vi "Frequency_Response_Data_Smoothing_Shifting_mV.vi"(0 "smoothing":bool, 1 "curveShifting":bool, 2 "Parameters.RefAmplitude":dbl, 3 "Parameters.UUTResponseLevel.frequency":dbl[](array[numeric]), 4 "Parameters.UUTResponseLevel.amplitude":dbl[](array[numeric]), 5 "FG.FrequencyLists.FrequencyResponse_LimitHigh.amplitude":dbl[](array[numeric]), 7 "FG.FrequencyLists.FrequencyResponse_LimitLow.amplitude":dbl[](array[numeric])) -> (14 "ProcessedFrequencyResponse":dbl[](array[numeric]))   [LabVIEW 2018]
uses:
  <vilib>/Analysis/6fits.llb/Curve Fitting Criteria.ctl
  <vilib>/Analysis/6fits.llb/General Linear Fit Algorithm.ctl
  <vilib>/Analysis/NI_AALPro.lvlib
panel:
  out "XY Graph 2":cluster{dbl[], dbl[]}[](graph)
  out "max value":dbl=0.5912174990705221
  out "min value":dbl=2.180066627082418
  out "ShiftCurveBy":dbl=1.38564206307647
  out "XY Graph":cluster{dbl[], dbl[]}[](graph)
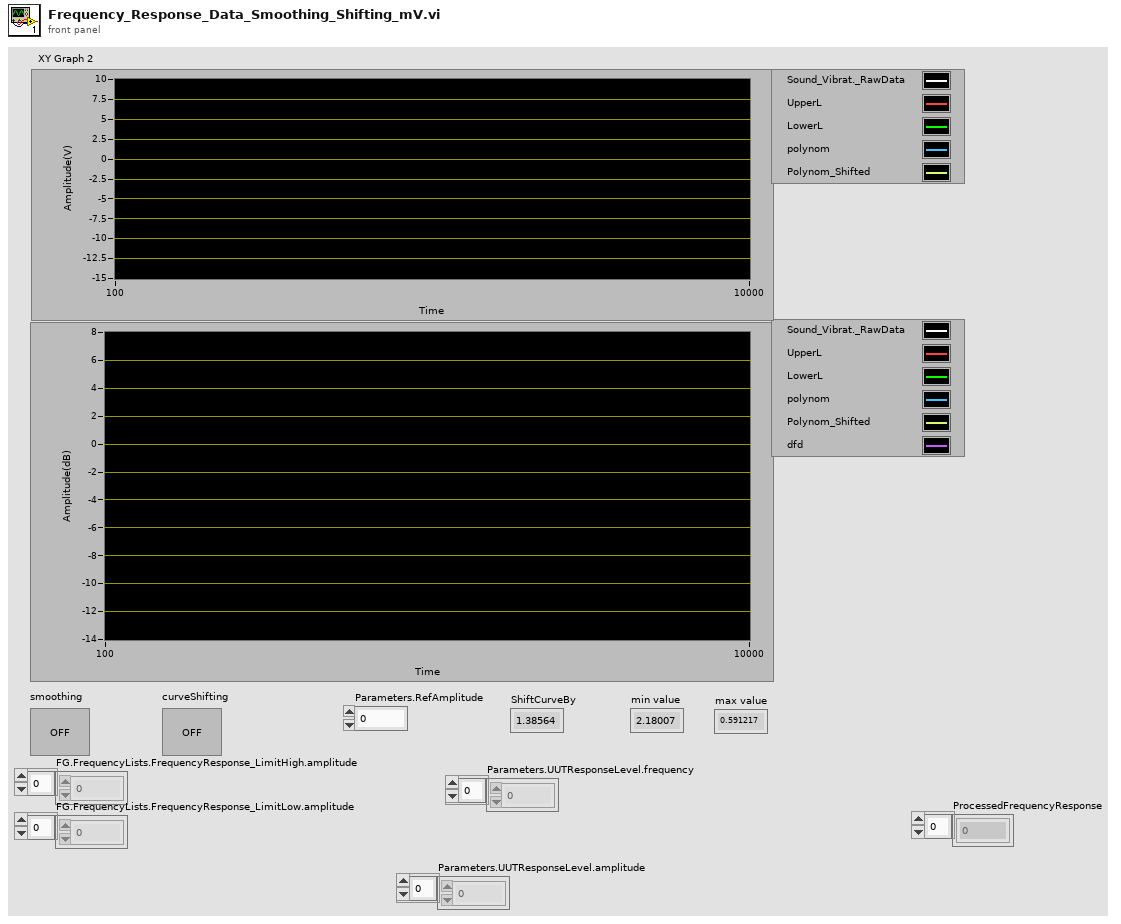
[diagram p1: front panel]
types:
  T1 = typedef "NI_AALPro.lvlib/General Linear Fit Algorithm.ctl" = u16
  T2 = typedef "NI_AALPro.lvlib/Curve Fitting Criteria.ctl" = u16
  T3 = cluster{"Parameters.UUTResponseLevel.frequency":dbl[], dbl[]}
  T4 = cluster{"Parameters.UUTResponseLevel.frequency":dbl[], dbl[]}[]
  T5 = cluster{"Parameters.UUTResponseLevel.frequency":dbl[], "FG.FrequencyLists.FrequencyResponse_LimitHigh.amplitude":dbl[]}
  T6 = cluster{"Parameters.UUTResponseLevel.frequency":dbl[], "FG.FrequencyLists.FrequencyResponse_LimitLow.amplitude":dbl[]}
  T7 = cluster{"Parameters.UUTResponseLevel.frequency":dbl[], "Best Polynomial Fit":dbl[]}
  T8 = cluster{"Parameters.UUTResponseLevel.frequency":dbl[], "Best Polynomial Fit":dbl[]}[]
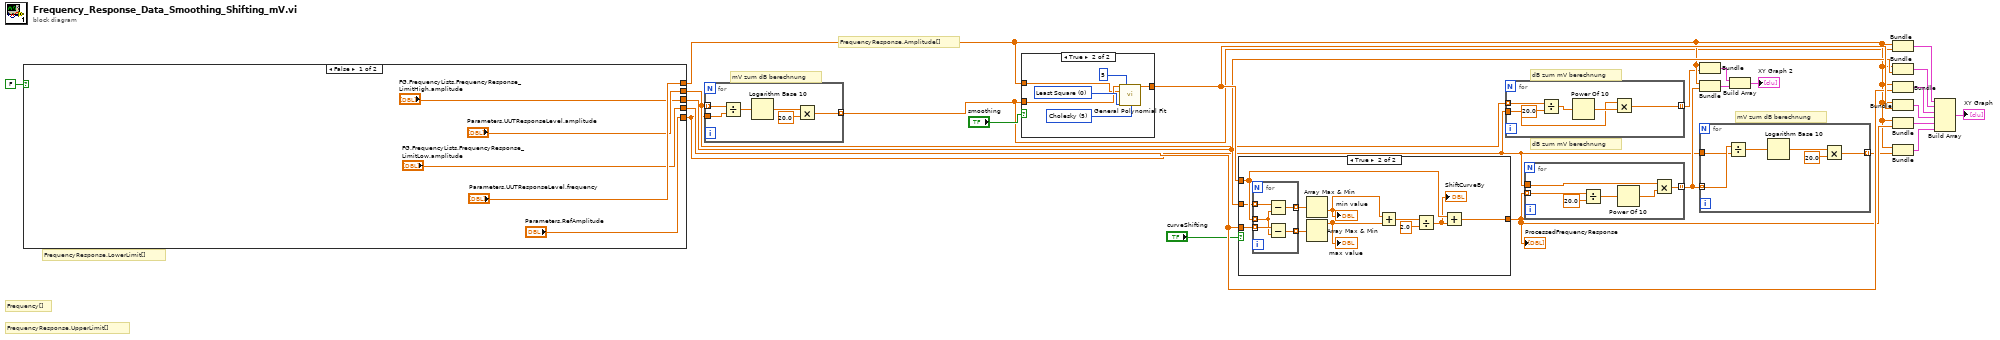
[diagram p0: block diagram]
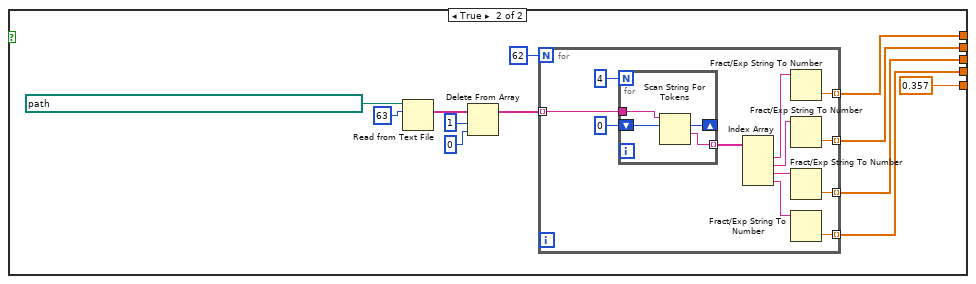
[diagram p2: hidden frame]
diagram:
  # "mV zum dB berechnung"
  # "mV zum dB berechnung"
  # "dB zum mV berechnung"
  # "dB zum mV berechnung"
  # "FrequencyResponse.LowerLimit[]"
  # "FrequencyResponse.UpperLimit[]"
  # "FrequencyResponse.Amplitude[]"
  # "Frequency[]"
  n1 = case shown="False" FALSE {
    tunnel: ["FG.FrequencyLists.FrequencyResponse_LimitLow.amplitude" w34] -> w17
    tunnel: ["FG.FrequencyLists.FrequencyResponse_LimitHigh.amplitude" w33] -> w16
    tunnel: ["Parameters.UUTResponseLevel.amplitude" w32] -> w3
    tunnel: ["Parameters.UUTResponseLevel.frequency" w31] -> w8
    tunnel: ["Parameters.RefAmplitude" 0.357 ("Parameters.RefAmplitude")] -> w2
    frame False {
    }
    frame True {
      n2 = Read from Text File(file (use dialog)=path "C:/Users/vr.ext/Desktop/Smoothing FG/SVT_Prüfstand_FG.txt", count=63) -> (text=w38:string[])  [unwired: 2 in, 3 out]
      n3 = Delete From Array(array=w38, length=1, index=0) -> (array with subset deleted=w35:string[])  [unwired: 1 out]
      n4 = for {
        N: 62 -> [_]
        tunnel: w35 -> [w51] mode=indexing
        tunnel: [w53] -> w31 mode=indexing
        tunnel: [w52] -> w32 mode=indexing
        tunnel: [w43] -> w33 mode=indexing
        tunnel: [w42] -> w34 mode=indexing
        n5 = for {
          N: 4 -> [_]
          tunnel: w51 -> [w56]
          shift-right: [w57] -> _
          shift-left: 0 ("count") -> [w55]
          tunnel: [w54] -> w49 mode=indexing
          n6 = Scan String For Tokens(8:w55, 9:w56) -> (1:w54:string, 2:w57:i32)  [unwired: 4 in, 2 out]
        }
        n7 = Index Array(array=w49) -> (element #1=w48:string, element #2=w47:string, element #3=w45:string, element #4=w44:string)  [unwired: 4 in]
        n8 = Fract/Exp String To Number(string=w48) -> (number=w53:dbl)  [unwired: 3 in, 1 out]
        n9 = Fract/Exp String To Number(string=w47) -> (number=w52:dbl)  [unwired: 3 in, 1 out]
        n10 = Fract/Exp String To Number(string=w45) -> (number=w43:dbl)  [unwired: 3 in, 1 out]
        n11 = Fract/Exp String To Number(string=w44) -> (number=w42:dbl)  [unwired: 3 in, 1 out]
      }
    }
  }
  n12 = for {
    tunnel: w3 -> [w62] mode=indexing
    tunnel: [w59] -> w1 mode=indexing
    tunnel: w2 -> [w58]
    n13 = Divide(x=w62, y=w58) -> (x/y=w61:dbl)
    n14 = Logarithm Base 10(1:w61) -> (0:w60:dbl)
    n15 = Multiply(x=w60, y=20.0) -> (x*y=w59:dbl)
  }
  n16 = case shown="True" "smoothing" {
    tunnel: w1 -> [w64 w67]
    tunnel: w8 -> [_ w66]
    tunnel: [w64 w65] -> w19
    frame False {
    }
    frame True {
      w69 = T1 5 items=["SVD", "Givens", "Givens2", "Householder", "LU Decomposition", "Cholesky", "SVD for Rank Deficient H"] ("algorithm")
      w70 = T2 0 items=["Least Square", "Least Absolute Residual", "Bisquare"] ("method")
      n17 = call <vilib>:"General Polynomial Fit.vi"("Y"=w67, "polynomial order"=5, "X"=w66, "method"=w70, "algorithm"=w69) -> ("Best Polynomial Fit"=w65:dbl[])  [unwired: 7 in, 3 out]
    }
  }
  n18 = case shown="True" "curveShifting" {
    tunnel: w19 -> [w71 w80]
    tunnel: [w71 w79] -> w11
    tunnel: w17 -> [_ w78]
    tunnel: w16 -> [_ w77]
    frame False {
    }
    frame True {
      n19 = for {
        tunnel: w77 -> [w87] mode=indexing
        tunnel: w80 -> [w84] mode=indexing
        tunnel: [w86] -> w82 mode=indexing
        tunnel: w78 -> [w85] mode=indexing
        tunnel: [w83] -> w81 mode=indexing
        n20 = Subtract(x=w87, y=w84) -> (x-y=w86:dbl)
        n21 = Subtract(x=w85, y=w84) -> (x-y=w83:dbl)
      }
      n22 = Array Max & Min(array=w82) -> (min value=w76:dbl)  [unwired: 3 out]
      "min value" <- w76
      n23 = Array Max & Min(array=w81) -> (max value=w75:dbl)  [unwired: 3 out]
      "max value" <- w75
      n24 = Add(x=w76, y=w75) -> (x+y=w74:dbl)
      n25 = Divide(x=w74, y=2.0) -> (x/y=w72:dbl)
      "ShiftCurveBy" <- w72
      n26 = Add(x=w80, y=w72) -> (x+y=w79:dbl[])
    }
  }
  "ProcessedFrequencyResponse" <- w11
  n27 = for {
    tunnel: w3 -> [w93] mode=indexing
    tunnel: [w89] -> w4 mode=indexing
    tunnel: w2 -> [w88]
    n28 = Divide(x=w93, y=20.0) -> (x/y=w91:dbl)
    n29 = Power Of 10(x=w91) -> (10^x=w90:dbl)
    n30 = Multiply(x=w88, y=w90) -> (x*y=w89:dbl)
  }
  n31 = for {
    tunnel: w11 -> [w99] mode=indexing
    tunnel: [w95] -> w9 mode=indexing
    tunnel: w2 -> [w94]
    n32 = Divide(x=w99, y=20.0) -> (x/y=w97:dbl)
    n33 = Power Of 10(x=w97) -> (10^x=w96:dbl)
    n34 = Multiply(x=w94, y=w96) -> (x*y=w95:dbl)
  }
  n35 = Bundle("Parameters.UUTResponseLevel.frequency"=w8, w4) -> (w12:T3)  [unwired: 1 in]
  n36 = Bundle("Parameters.UUTResponseLevel.frequency"=w8, w9) -> (w10:T3)  [unwired: 1 in]
  n37 = for {
    tunnel: w9 -> [w104] mode=indexing
    tunnel: [w101] -> w7 mode=indexing
    tunnel: w2 -> [w100]
    n38 = Divide(x=w104, y=w100) -> (x/y=w103:dbl)
    n39 = Logarithm Base 10(1:w103) -> (0:w102:dbl)
    n40 = Multiply(x=w102, y=20.0) -> (x*y=w101:dbl)
  }
  n41 = Build Array(w12, w10) -> (→"XY Graph 2":T4)
  n42 = Bundle("Parameters.UUTResponseLevel.frequency"=w8, w1) -> (w22:T3)  [unwired: 1 in]
  n43 = Bundle("Parameters.UUTResponseLevel.frequency"=w8, "FG.FrequencyLists.FrequencyResponse_LimitHigh.amplitude"=w16) -> (w21:T5)  [unwired: 1 in]
  n44 = Bundle("Parameters.UUTResponseLevel.frequency"=w8, "FG.FrequencyLists.FrequencyResponse_LimitLow.amplitude"=w17) -> (w20:T6)  [unwired: 1 in]
  n45 = Bundle("Parameters.UUTResponseLevel.frequency"=w8, "Best Polynomial Fit"=w19) -> (w23:T7)  [unwired: 1 in]
  n46 = Bundle("Parameters.UUTResponseLevel.frequency"=w8, "Best Polynomial Fit"=w11) -> (w18:T7)  [unwired: 1 in]
  n47 = Bundle("Parameters.UUTResponseLevel.frequency"=w8, w7) -> (w6:T3)  [unwired: 1 in]
  n48 = Build Array(w22, w21, w20, w23, w18, w6) -> (→"XY Graph":T8)
